vi "macro_Ctrl_RamseteExecute.vi"() -> ()   [LabVIEW 2019]
uses:
  <vilib>/Rock Robotics/WPI/ThirdParty/JAS_Junk/TrajLib/Trajectory_Library.lvlib
  <vilib>/Rock Robotics/WPI/ThirdParty/JAS_Junk/TrajLib/TypeDef/TRANSLATION2D.ctl
  <vilib>/Rock Robotics/WPI/ThirdParty/JAS_Junk/TrajLib/TypeDef/ROTATION2D.ctl
  <vilib>/Rock Robotics/WPI/ThirdParty/JAS_Junk/TrajLib/TypeDef/POSE2D.ctl
  TypeDef/PathPlannerPathConstraints.ctl
  TypeDef/PathPlannerTrajectoryState.ctl
panel:
  out "Left Speed Dmd M/S":dbl
  out "Right Speed Dmd M/S":dbl
  in  "Reset":bool
  in  "PathPlannerState":T1={"TimeSeconds"=0.0, "VelocityMPS"=0.0, "AccerationMpsSq"=0.0, "HeadingAngularVelRadPerSec"=0.0, "PositionMeters"={"X"=0.0, "Y"=0.0}, "Heading"={"VALUE"=0.0, "COS"=1.0, "SIN"=0.0}, "TargetHolonomicRotation"={"VALUE"=0.0, "COS"=1.0, "SIN"=0.0}, "CurvatureRadPerMeter"=0.0, "PathPlannerConstraints"={"MaxVelocityMps;"=0.0, "MaxAccelerationMpsSq;"=0.0, "MaxAngularVelRadPsEc;"=0.0, "MaxAngularAccRadPSecSq"=0.0, "Exists"=FALSE}, "DeltaPos"=0.0} {"TargetHolonomicRotation"."SIN" format="%13.4f"; "TargetHolonomicRotation"."COS" format="%13.4f"; "TargetHolonomicRotation"."VALUE" format="%13.4f"; "Heading"."SIN" format="%13.4f"; "Heading"."COS" format="%13.4f"; "Heading"."VALUE" format="%13.4f"; "PositionMeters"."Y" format="%14.3f"; "PositionMeters"."X" format="%14.3f"}
  in  "currentPose":T5={"TRANSLATION"={"X"=0.0, "Y"=0.0}, "ROTATION"={"VALUE"=0.0, "COS"=1.0, "SIN"=0.0}} {"ROTATION"."SIN" format="%13.4f"; "ROTATION"."COS" format="%13.4f"; "ROTATION"."VALUE" format="%13.4f"; "TRANSLATION"."Y" format="%14.3f"; "TRANSLATION"."X" format="%14.3f"}
  out "Position Error M":dbl
  out "At Reference":bool
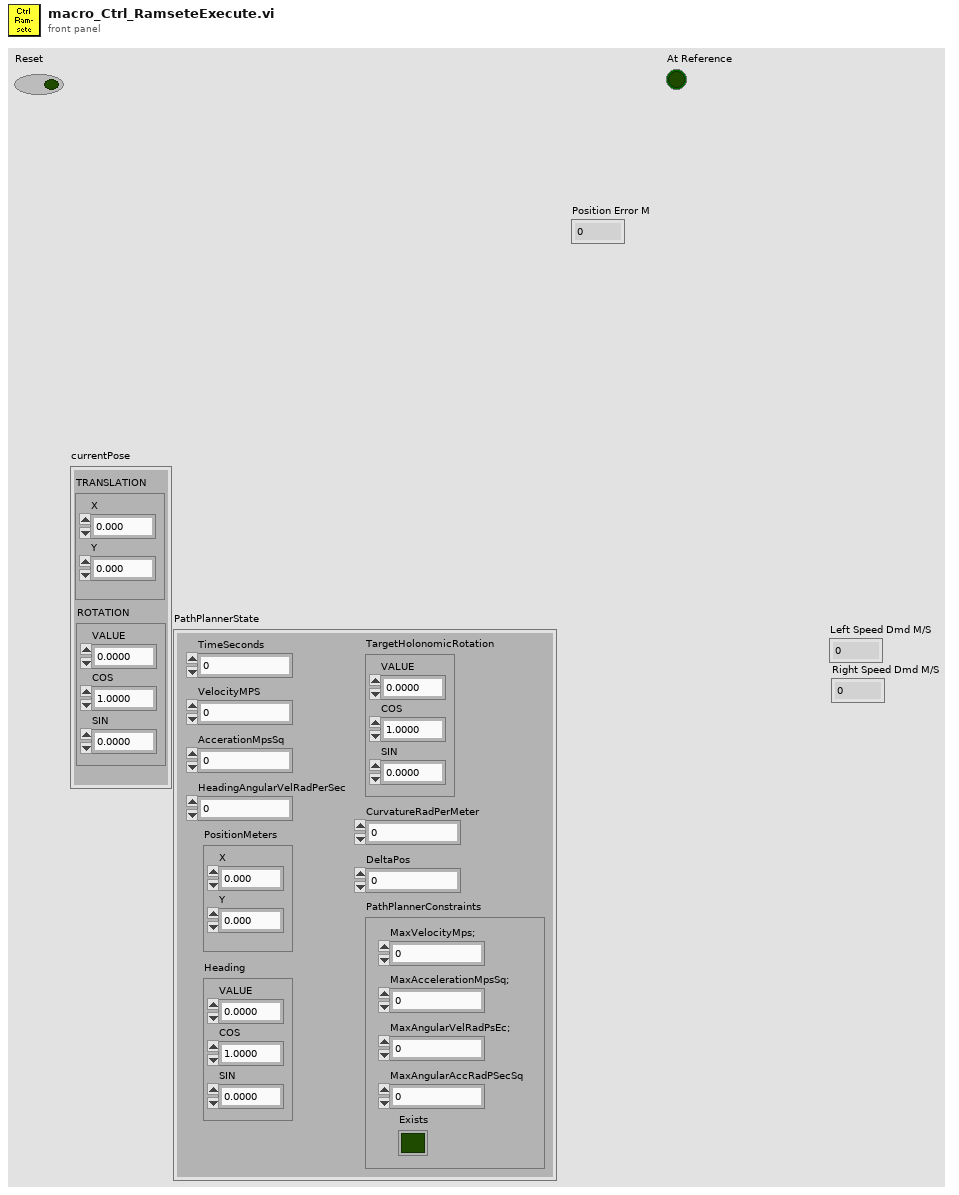
[diagram p1: front panel]
types:
  T1 = typedef "PathPlannerTrajectoryState.ctl" = cluster{"TimeSeconds":dbl, "VelocityMPS":dbl, "AccerationMpsSq":dbl, "HeadingAngularVelRadPerSec":dbl, "PositionMeters":T2, "Heading":T3, "TargetHolonomicRotation":T3, "CurvatureRadPerMeter":dbl, "PathPlannerConstraints":T4, "DeltaPos":dbl}
  T2 = typedef "Trajectory_Library.lvlib/TRANSLATION2D.ctl" = cluster{"X":dbl, "Y":dbl}
  T3 = typedef "Trajectory_Library.lvlib/ROTATION2D.ctl" = cluster{"VALUE":dbl, "COS":dbl, "SIN":dbl}
  T4 = typedef "PathPlannerPathConstraints.ctl" = cluster{"MaxVelocityMps;":dbl, "MaxAccelerationMpsSq;":dbl, "MaxAngularVelRadPsEc;":dbl, "MaxAngularAccRadPSecSq":dbl, "Exists":bool}
  T5 = typedef "Trajectory_Library.lvlib/POSE2D.ctl" = cluster{"TRANSLATION":T2, "ROTATION":T3}
  T6 = typedef "Trajectory_Library.lvlib/RAMSETE_EXE_TUNING.ctl" = cluster{"B":dbl, "Zeta":dbl, "X Tolerance M":dbl, "Y Tolerance M":dbl, "Heading Tolerance RAD":dbl, "Track Width M":dbl, "Max Speed M/S":dbl}
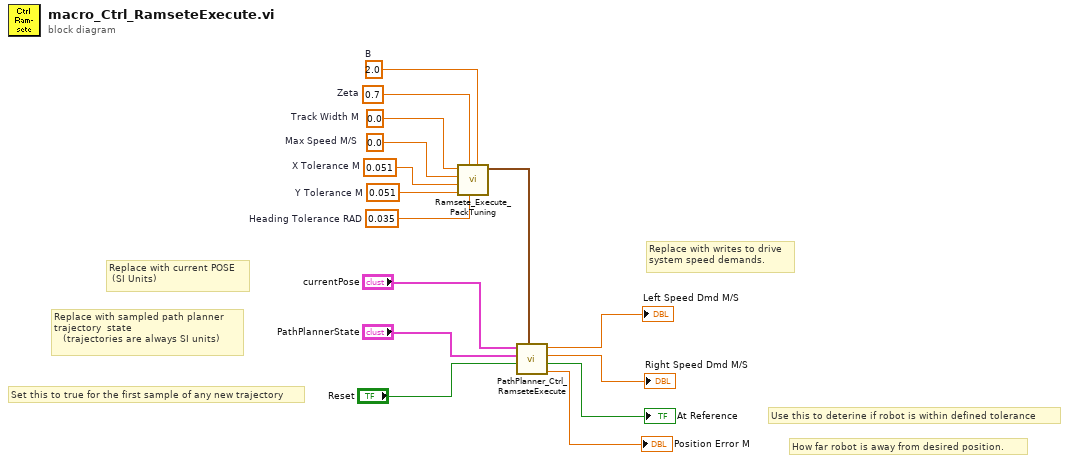
[diagram p0: block diagram]
diagram:
  w15 = 0.0  # Track Width M
  w14 = 0.0  # Max Speed M/S
  w13 = 0.051  # X Tolerance M
  w12 = 0.051  # Y Tolerance M
  w11 = 0.7  # Zeta
  w10 = 0.035  # Heading Tolerance RAD
  w9 = 2.0  # B
  # "Replace with writes to drive\nsystem speed demands."
  # "Replace with current POSE\n (SI Units)"
  # "Replace with sampled path planner \ntrajectory  state \n   (trajectories are always SI units)"
  # "How far robot is away from desired position."
  # "Use this to deterine if robot is within defined tolerance"
  # "Set this to true for the first sample of any new trajectory"
  n1 = call <vilib>:"Ramsete_Execute_PackTuning.vi"("B"=w9, "Heading Tolerance RAD"=w10, "Zeta"=w11, "Y Tolerance M"=w12, "X Tolerance M"=w13, "Max Speed M/S"=w14, "Track Width M"=w15) -> ("RAMSETE_EXE_TUNING"=w8:T6)  [unwired: 4 in]
  n2 = call "PathPlanner_Ctrl_RamseteExecute.vi"("RAMSETE_EXE_TUNING SI"=w8, "Reset"="Reset", "PathPlannerState"="PathPlannerState", "Current Pose SI"="currentPose") -> ("Position Error M"=→"Position Error M":dbl, "At Reference"=→"At Reference":bool, "Right Speed Dmd M/S"=→"Right Speed Dmd M/S":dbl, "Left Speed Dmd M/S"=→"Left Speed Dmd M/S":dbl)  [unwired: 3 in, 1 out]
